vi "easy stream start U3.vi"(4 "PC buffer size (seconds)":dbl=10.0 format="%.2f", 6 "Scan List (-)":u8[](array[numeric])=[31, 31, 31, 31, 31, 31, 31, 31, 31, 31, 31, 31, 31, 31, 31, 31, 31, 31, 31, 31, 31, 31, 31, 31, 31, 31, 31, 31, 31, 31, 31, 31, 31, 31, 31, 31, 31, 31, 31, 31, 31, 31, 31, 31, 31, 31, 31, 31, 31, 31, 31, 31, 31, 31, 31, 31, 31, 31, 31, 31, 31, 31, 31, 31, 31, 31, 31, 31, 31, 31, 31, 31, 31, 31, 31, 31, 31, 31, 31, 31, 31, 31, 31, 31, 31, 31, 31, 31, 31, 31, 31, 31, 31, 31, 31, 31, 31, 31, 31, 31, 31, 31, 31, 31, 31, 31, 31, 31, 31, 31, 31, 31, 31, 31, 31, 31, 31, 31, 31, 31, 31, 31, 31, 31, 31, 31, 31, 31], 7 "Device Info":T1={"DeviceType"=3, "Connection Type"=0, "Address"="1", "FirstFound"=TRUE} {"Connection Type" items=["USB", "Ethernet"]}, 8 "error in":errorcluster, 9 "Scan List (+)":u8[](array[numeric])=[0, 1, 2, 3], 10 "Scan Rate (Hz)":dbl=1000.0 format="%.3f") -> (0 "error out":errorcluster, 1 "# Channels":i32, 2 "Actual Scan Rate (Hz)":dbl=1000.0 format="%.3f", 3 "Handle Out":i32)   [LabVIEW 2020]
panel:
  # "By default, this VI configures the\ndevice for \"WAIT\" stream read mode.\n\nScan List (-) only needed if doing something\nbesides single-ended channels."
  # "3 = U3\n6 = U6\n9 = UE9"
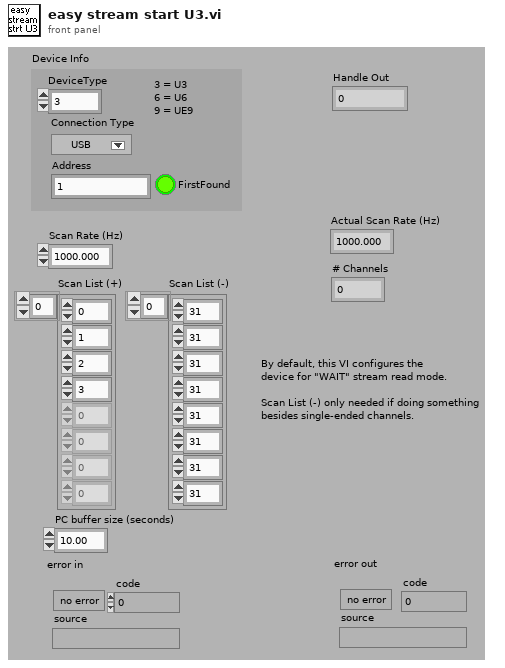
[diagram p1: front panel]
types:
  T1 = cluster{"DeviceType":i32, "Connection Type":u16, "Address":string, "FirstFound":bool}
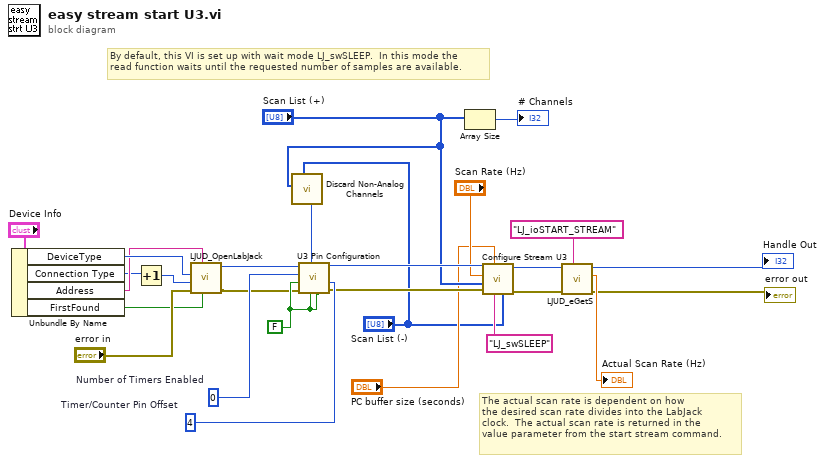
[diagram p0: block diagram]
diagram:
  w21 = FALSE ("Enable DAC1")
  w26 = u8 0  # Number of Timers Enabled
  w27 = u8 4  # Timer/Counter Pin Offset
  # "By default, this VI is set up with wait mode LJ_swSLEEP.  In this mode the\nread function waits until the requested number of samples are available."
  # "The actual scan rate is dependent on how\nthe desired scan rate divides into the LabJack\nclock.  The actual scan rate is returned in the\nvalue parameter from the start stream command."
  n1 = Unbundle By Name("Device Info") -> ("DeviceType"=w8:i32, "Connection Type"=w4:u16, "Address"=w6:string, "FirstFound"=w5:bool)
  n2 = Increment(x=w4) -> (x+1=w3:u16)
  n3 = call "LJUD_OpenLabJack.vi"("FirstFound"=w5, "Address"=w6, "error in"="error in", "ConnectionType"=w3, "DeviceType"=w8) -> ("error out"=w20:errorcluster, "Handle"=w19:i32)  [unwired: 5 in]
  n4 = call "Discard Non-Analog Channels.vi"("Channels In (-)"="Scan List (-)", "Channels In"="Scan List (+)") -> ("FIO/EIO Analog Enable"=w22:i32)  [unwired: 6 in, 3 out]
  n5 = call "U3 Pin Configuration.vi"("Timer/Counter Pin Offset"=w27, "Enable Counter1"=w21, "Enable Counter0"=w21, "FIO/EIO Analog Enable"=w22, "error in"=w20, "Enable DAC1"=w21, "Number of Timers Enabled"=w26, "Handle In"=w19) -> ("error out"=w25:errorcluster, "Handle Out"=w24:i32)  [unwired: 2 in]
  n6 = Array Size(array="Scan List (+)") -> (size(s)=→"# Channels":i32)
  n7 = call "Configure Stream U3.vi"("Scan List (-)"="Scan List (-)", "Wait Mode"="LJ_swSLEEP" ("Wait Mode (2)"), "PC buffer size (seconds)"="PC buffer size (seconds)", "error in"=w25, "Scan List (+)"="Scan List (+)", "Scan Rate (Hz)"="Scan Rate (Hz)", "Handle In"=w24) -> ("error out"=w15:errorcluster, "Handle Out"=w14:i32)  [unwired: 2 in, 1 out]
  n8 = call "LJUD_eGetS.vi"("IOType"="LJ_ioSTART_STREAM", "error in"=w15, "Handle In"=w14) -> ("error out"=→"error out":errorcluster, "Value Read"=→"Actual Scan Rate (Hz)":dbl, "Handle Out"=→"Handle Out":i32)  [unwired: 6 in]
